vi "MCL Release Handle.vi"(11 "handle":i32) -> ()   [LabVIEW 2017, in "Madlib.lvlib"]
doc: "MADLIB_API void MCL_ReleaseHandle(int handle);"
uses:
  Madlib.lvlib
  Madlib.dll
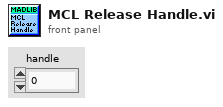
[diagram p1: front panel]
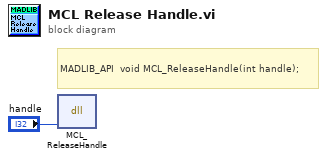
[diagram p0: block diagram]
diagram:
  # "MADLIB_API  void\tMCL_ReleaseHandle(int handle);"
  n1 = dll-call lib="C:/Users/francesco/dev/pump-probe/Piezo/lvlib/Madlib.*" fn="MCL_ReleaseHandle"("handle"="handle") -> ()  [unwired: 5 in, 2 out]
